vi "Read configDirectoryPathWindows.vi"(8 "error in (no error)":errorcluster, 11 "ComponentData in":refnum<class "ComponentData.lvclass">) -> (0 "error out":errorcluster, 2 "configDirectoryPathWindows":path, 3 "ComponentData out":refnum<class "ComponentData.lvclass">)   [LabVIEW 2013, in "ComponentData.lvlib" / "ComponentData.lvclass"]
uses:
  <userlib>/Common/Component/Application/RT/ComponentData/ComponentData/ComponentData.lvclass
  <userlib>/Common/Component/Application/RT/ComponentData/ComponentData/ComponentData.lvclass/ComponentData.ctl
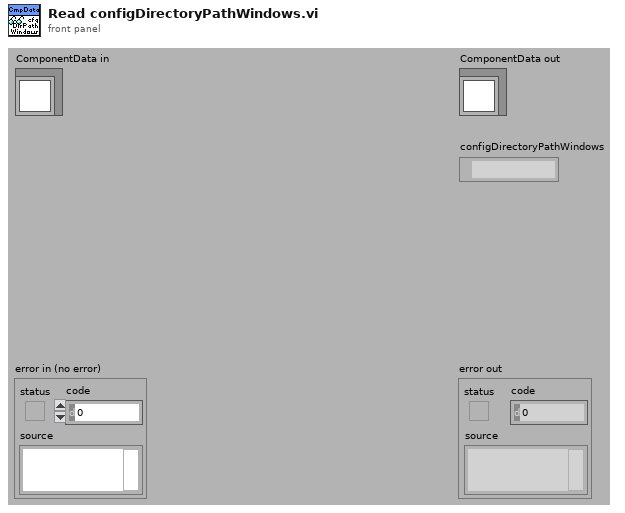
[diagram p1: front panel]
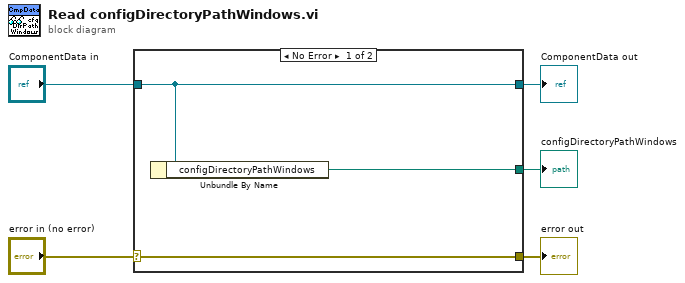
[diagram p0: block diagram]
diagram:
  n1 = case shown="No Error" "error in (no error)" {
    selector: "error in (no error)" -> [w8 w9]
    tunnel: [w8 w9] -> w4
    tunnel: [w7 w10] -> w2
    tunnel: "ComponentData in" -> [w7 w10]
    tunnel: [w6 _] -> w1
    frame No Error {
      n2 = Unbundle By Name(w7) -> ("configDirectoryPathWindows"=w6:path)
    }
    frame Error {
    }
  }
  "error out" <- w4
  "ComponentData out" <- w2
  "configDirectoryPathWindows" <- w1
